vi "DHE_GetexposureID.vi"(8 "error in (no error)":errorcluster, 10 "UT in":string) -> (0 "error out":errorcluster, 2 "expID":string)   [LabVIEW 2016]
uses:
  DBSHAND/private/vis/DatabaseHand_Element_Get(bool).vi
  DBSHAND/private/vis/DatabaseHand_Element_Get(string).vi
  DBSHAND/private/vis/DatabaseHand_Element_Get(U32).vi
  DBSHAND/private/vis/DatabaseHand_Element_Set(string).vi
  DBSHAND/private/vis/DatabaseHand_Element_Set(U32).vi
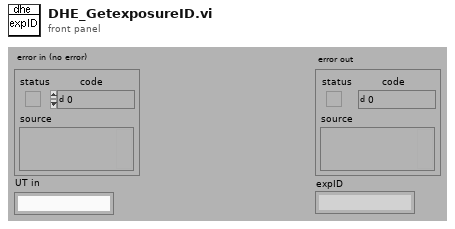
[diagram p1: front panel]
types:
  T1 = typedef "DatabaseHand_RefNum.ctl" = refnum<vi>
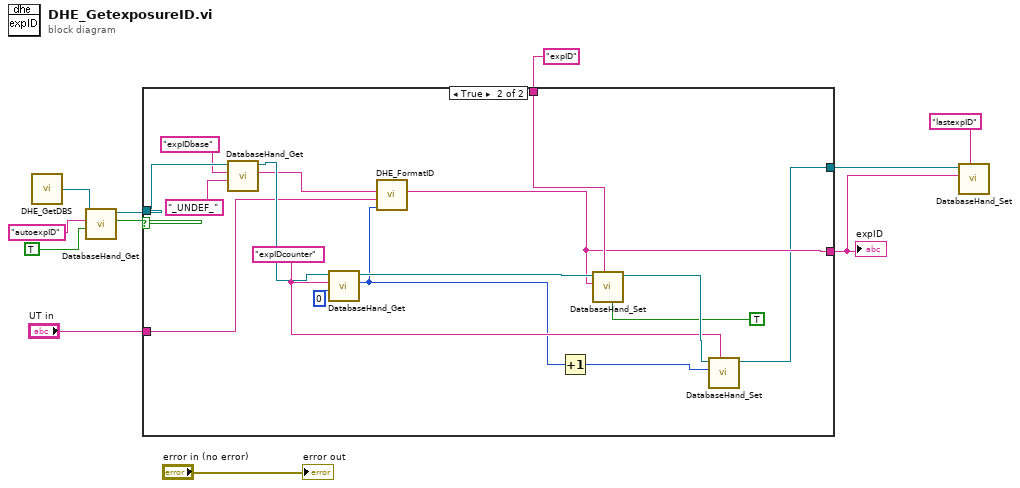
[diagram p0: block diagram]
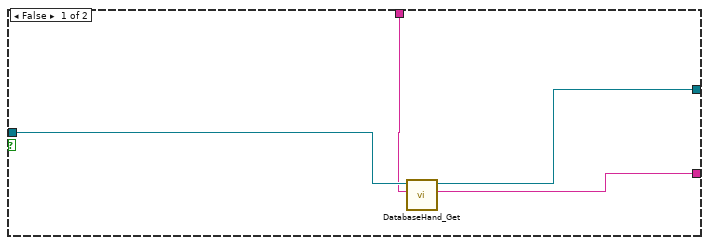
[diagram p2: hidden frame]
diagram:
  n1 = call "DHE_GetDBS.vi"() -> ("DHE_DBSRef"=w11:T1)  [unwired: 9 out]
  n2 = call-poly "DatabaseHand_Get.vi"("default value"=TRUE, "name"="autoexpID", "Database RefNum in"=w11) -> ("value"=w8:bool, "Database RefNum out"=w7:T1)  [unwired: 2 in, 5 out]
  n3 = case shown="True" w8 {
    tunnel: w7 -> [w15 w31]
    tunnel: [w13 w17] -> w1
    tunnel: "expID" ("name") -> [w14 w22]
    tunnel: "UT in" -> [_ w19]
    tunnel: [w12 w16] -> w2
    frame False {
      n4 = call-poly "DatabaseHand_Get.vi"("name"=w14, "Database RefNum in"=w15) -> ("value"=w13:string, "Database RefNum out"=w12:T1)  [unwired: 3 in, 5 out]
    }
    frame True {
      w25 = "expIDcounter" ("name")
      n5 = call-poly "DatabaseHand_Get.vi"("default value"="_UNDEF_", "name"="expIDbase", "Database RefNum in"=w31) -> ("value"=w20:string, "Database RefNum out"=w23:T1)  [unwired: 2 in, 5 out]
      n6 = call-poly "DatabaseHand_Get.vi"("default value"=u32 0 ("input 1"), "name"=w25, "Database RefNum in"=w23) -> ("value"=w18:u32, "Database RefNum out"=w28:T1)  [unwired: 2 in, 5 out]
      n7 = call "DHE_FormatID.vi"("id counter in"=w18, "UT in"=w19, "IDbase in"=w20) -> ("expID out"=w17:string)  [unwired: 8 out]
      n8 = Increment(x=w18) -> (x+1=w24:u32)
      n9 = call-poly "DatabaseHand_Set.vi"("enqueue? (F)"=TRUE, "name"=w22, "value"=w17, "Database RefNum in"=w28) -> ("Database RefNum out"=w26:T1)  [unwired: 4 in, 3 out]
      n10 = call-poly "DatabaseHand_Set.vi"("name"=w25, "value"=w24, "Database RefNum in"=w26) -> ("Database RefNum out"=w16:T1)  [unwired: 5 in, 3 out]
    }
  }
  "expID" <- w1
  n11 = call-poly "DatabaseHand_Set.vi"("name"="lastexpID", "value"=w1, "Database RefNum in"=w2) -> ()  [unwired: 5 in, 4 out]
  "error out" <- "error in (no error)"
